vi "Command Run MP.vi"(7 "Startup":bool) -> (0 "Parameter 2":dbl, 1 "Parameter 1":dbl, 2 "Reinitialize":bool, 3 "Completed":bool)   [LabVIEW 2017]
uses:
  Command Execution State.ctl
  Drive/Drive Globals.vi
  Globals/Position Data.vi
  <vilib>/Utility/file.llb/Read Delimited Spreadsheet (DBL).vi
  <vilib>/Utility/file.llb/Read Delimited Spreadsheet (string).vi
panel:
  out "thetaError PID":T1(graph)
  in  "Path name":string
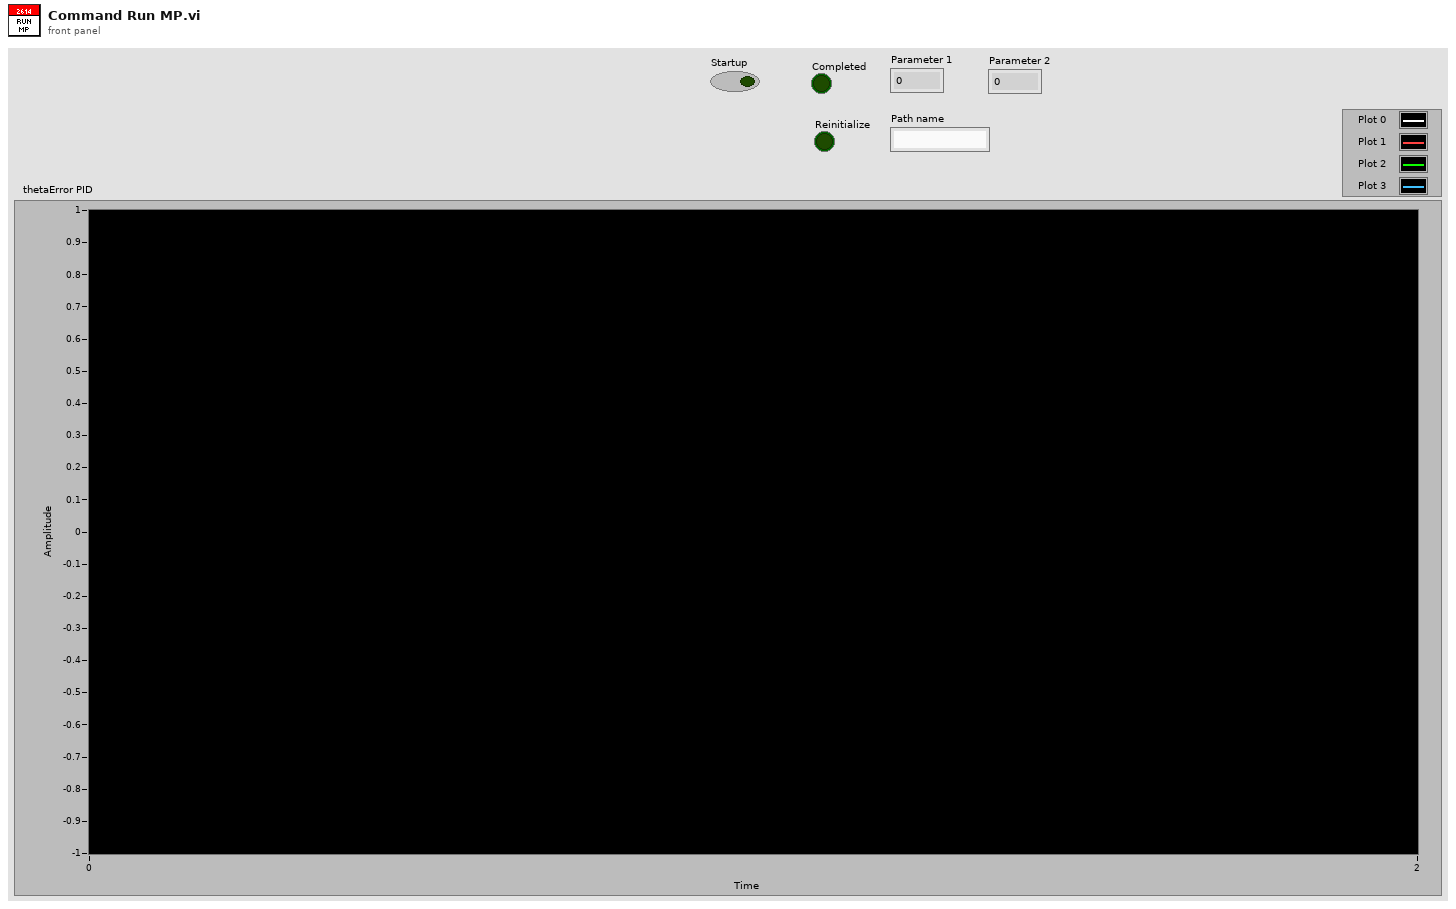
[diagram p1: front panel]
types:
  T1 = cluster{"Goal Wheel Position":dbl, dbl, "thetaError":dbl, "Command ":dbl}
  T2 = typedef "Command Execution State.ctl" = enum16{"Initialize", "Execute", "Finish"}
  T3 = cluster{"Goal Wheel Position":dbl, dbl, "Command ":dbl, "thetaError":dbl}
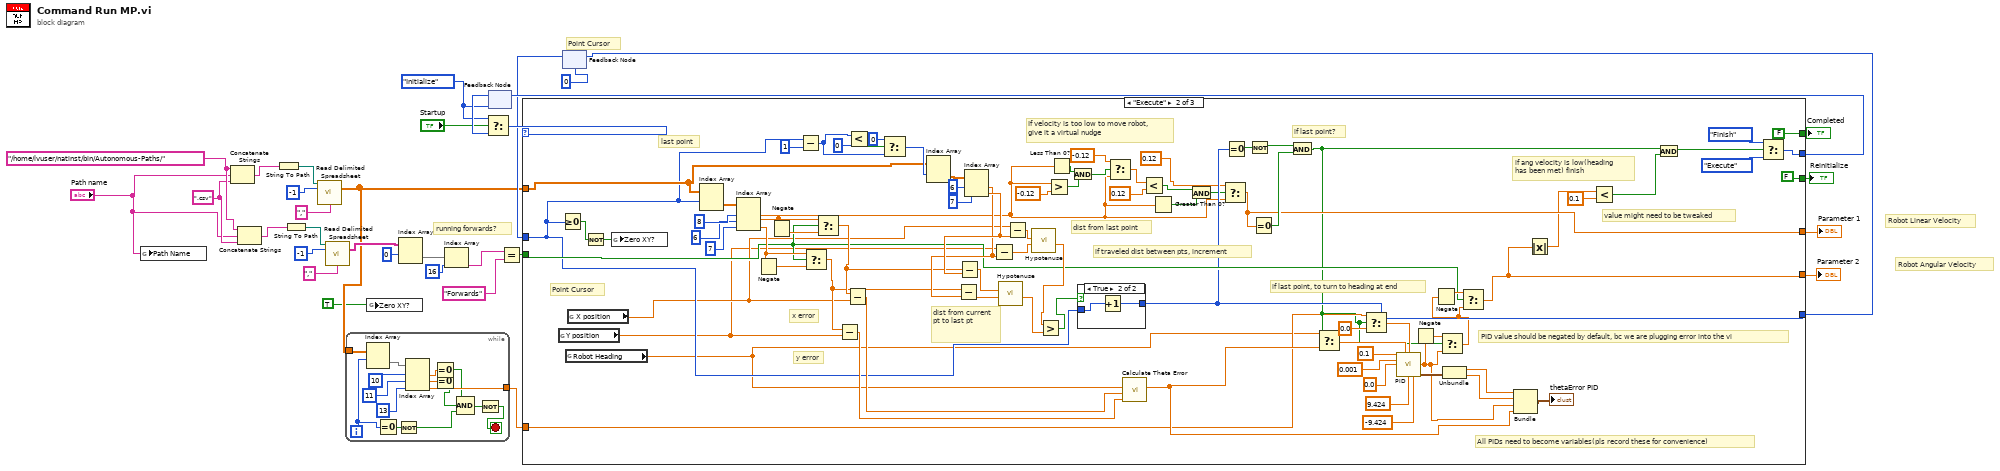
[diagram p0: block diagram]
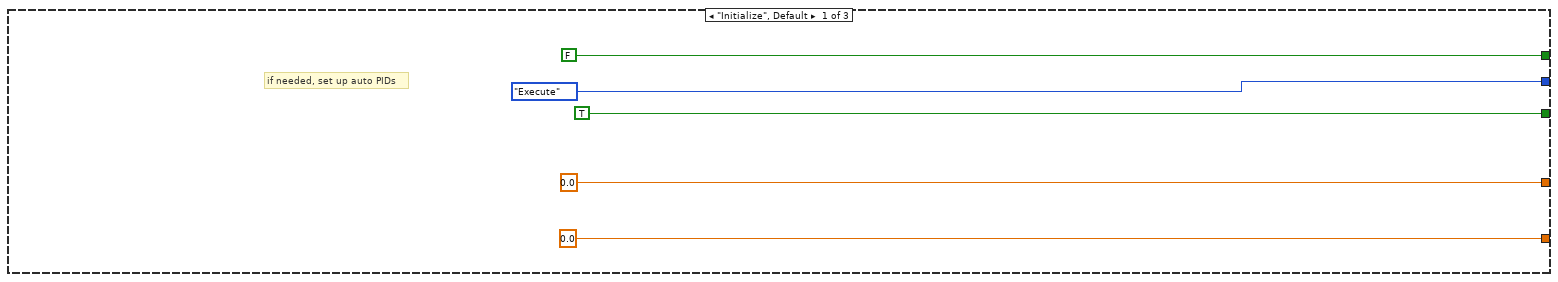
[diagram p2: hidden frame]
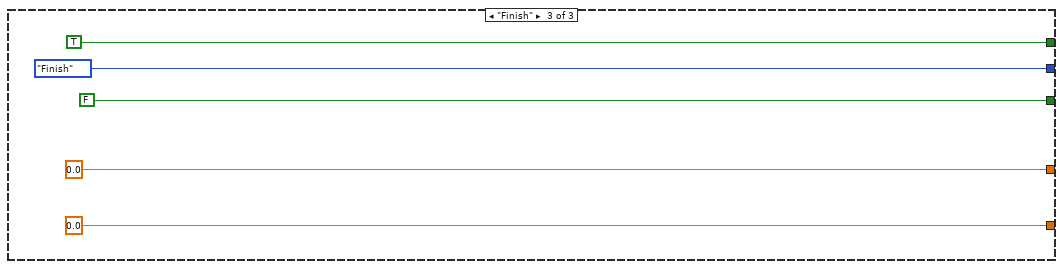
[diagram p4: hidden frame]
diagram:
  w12 = ".csv" ("string")
  w13 = "/home/lvuser/natinst/bin/Autonomous-Paths/"
  w28 = Command_Execution_State."Initialize" ("Play State")
  # "Point Cursor"
  # "running forwards?"
  # "Robot Angular Velocity"
  # "Robot Linear Velocity"
  n1 = global write "Position Data.vi" "Path Name"("Path name") -> ()
  n2 = Concatenate Strings(w13, "Path name", w12) -> (w22:string)
  n3 = Concatenate Strings(w13, "Path name", w12) -> (w16:string)
  n4 = String To Path(string=w22) -> (path=w21:path)
  n5 = String To Path(string=w16) -> (path=w17:path)
  n6 = call-poly <vilib>:"Read Delimited Spreadsheet.vi"("file path (dialog if empty)"=w21, "number of rows (all:-1)"=-1, "delimiter (\\t)"="," ("delimiter (\\t)")) -> ("all rows"=w3:dbl[][])  [unwired: 7 in, 5 out]
  n7 = call-poly <vilib>:"Read Delimited Spreadsheet.vi"("file path (dialog if empty)"=w17, "number of rows (all:-1)"=-1, "delimiter (\\t)"="," ("delimiter (\\t)")) -> ("all rows"=w11:string[][])  [unwired: 7 in, 5 out]
  n8 = while {
    tunnel: w3 -> [w48]
    tunnel: [w43] -> w2
    i -> [w40]
    stop <- w34 stop-if-true
    n9 = Index Array(array=w48, index (row)=w40) -> (element=w47:dbl[])  [unwired: 1 in]
    n10 = Equal To 0?(x=w40) -> (x = 0?=w39:bool)
    n11 = Not(x=w39) -> (.not. x?=w36:bool)
    n12 = Index Array(array=w47, index #1=10 ("index"), index #2=11 ("index"), index #3=13 ("index")) -> (element #1=w41:dbl, element #2=w42:dbl, element #3=w43:dbl)
    n13 = Equal To 0?(x=w41) -> (x = 0?=w37:bool)
    n14 = Equal To 0?(x=w42) -> (x = 0?=w38:bool)
    n15 = Compound Arithmetic op=AND(w37, w38, w36) -> (w35:bool)
    n16 = Not(x=w35) -> (.not. x?=w34:bool)
  }
  n17 = global write "Drive Globals.vi" "Zero XY?"(TRUE ("Zero XY?")) -> ()
  n18 = Index Array(array=w11, index (row)=0) -> (element=w20:string[])  [unwired: 1 in]
  n19 = Index Array(array=w20, index=16) -> (element=w10:string)
  n20 = feedback #1(w28) -> (w31:T2)
  n21 = Select(t=w28, s="Startup", f=w31) -> (s? t:f=w33:T2)
  n22 = Equal?(x=w10, y="Forwards") -> (x = y?=w8:bool)
  n23 = feedback #2(0 ("index")) -> (w6:i32)
  n24 = case shown="\"Execute\"" w33 {
    tunnel: [Command_Execution_State."Execute" ("Play State") w137 Command_Execution_State."Finish" ("Play State")] -> w32
    tunnel: [0.0 ("Back Left Spin Power") w72 0.0 ("Back Left Spin Power")] -> w30
    tunnel: [0.0 ("Front Right Spin Power") w63 0.0 ("Front Right Spin Power")] -> w29
    tunnel: [FALSE FALSE TRUE] -> w27
    tunnel: [TRUE FALSE FALSE] -> w26
    tunnel: w3 -> [_ w103 _]
    tunnel: w8 -> [_ w101 _]
    tunnel: w6 -> [_ w87 _]
    tunnel: [_ w85 _] -> w5
    tunnel: w2 -> [_ w68 _]
    frame "Initialize", Default {
      # "if needed, set up auto PIDs"
    }
    frame "Execute" {
      # "value might need to be tweaked"
      # "if ang velocity is low(heading\nhas been met) finish"
      # "if last point, to turn to heading at end"
      # "if last point?"
      # "PID value should be negated by default, bc we are plugging error into the vi"
      # "If velocity is too low to move robot,\ngive it a virtual nudge"
      # "if traveled dist between pts, increment"
      # "All PIDs need to become variables(pls record these for convenience)"
      # "dist from current pt to last pt"
      # "dist from last point"
      # "last point"
      # "y error"
      # "x error"
      # "Point Cursor"
      n25 = global read "Drive Globals.vi" "Y position"() -> (w54:dbl)
      n26 = Greater Or Equal To 0?(x=w87) -> (x >= 0?=w86:bool)
      n27 = global read "Drive Globals.vi" "Robot Heading"() -> (w56:dbl)
      n28 = global read "Drive Globals.vi" "X position"() -> (w55:dbl)
      n29 = Not(x=w86) -> (.not. x?=w57:bool)
      n30 = global write "Drive Globals.vi" "Zero XY?"(w57) -> ()
      n31 = Index Array(array=w103, index (row)=w87) -> (element=w132:dbl[])  [unwired: 1 in]
      n32 = Index Array(array=w132, index #1=8 ("index"), index #2=6 ("index"), index #3=7 ("index")) -> (element #1=w73:dbl, element #2=w108:dbl, element #3=w106:dbl)
      n33 = Negate(x=w106) -> (-x=w105:dbl)
      n34 = Negate(x=w108) -> (-x=w107:dbl)
      n35 = Subtract(x=w87, y=1) -> (x-y=w88:i32)
      n36 = Select(t=w106, s=w101, f=w105) -> (s? t:f=w104:dbl)
      n37 = Select(t=w108, s=w101, f=w107) -> (s? t:f=w109:dbl)
      n38 = Subtract(x=w104, y=w54) -> (x-y=w111:dbl)
      n39 = Subtract(x=w109, y=w55) -> (x-y=w110:dbl)
      n40 = Less?(x=w88, y=0) -> (x < y?=w115:bool)
      n41 = Select(t=0, s=w115, f=w88) -> (s? t:f=w112:i32)
      n42 = Index Array(array=w103, index (row)=w112) -> (element=w128:dbl[])  [unwired: 1 in]
      n43 = Index Array(array=w128, index #1=6 ("index"), index #2=7 ("index")) -> (element #1=w124:dbl, element #2=w125:dbl)
      n44 = Subtract(x=w104, y=w124) -> (x-y=w120:dbl)
      n45 = Subtract(x=w109, y=w125) -> (x-y=w121:dbl)
      n46 = Subtract(x=w54, y=w124) -> (x-y=w122:dbl)
      n47 = call "Hypotenuse.vi"("b"=w120, "a"=w121) -> ("c"=w119:dbl)  [unwired: 9 in]
      n48 = Subtract(x=w55, y=w125) -> (x-y=w123:dbl)
      n49 = call "Hypotenuse.vi"("b"=w122, "a"=w123) -> ("c"=w118:dbl)  [unwired: 9 in]
      n50 = Greater?(x=w118, y=w119) -> (0:w117:bool)
      n51 = Greater?(x=w73, y=-0.12) -> (0:w78:bool)
      n52 = Less Than 0?(x=w73) -> (x < 0?=w82:bool)
      n53 = And(x=w82, y=w78) -> (x .and. y?=w76:bool)
      n54 = case shown="True" w117 {
        tunnel: [w138 w140] -> w85
        tunnel: w87 -> [w138 w139]
        frame False {
        }
        frame True {
          n55 = Increment(x=w139) -> (x+1=w140:i32)
        }
      }
      n56 = Select(t=-0.12, s=w76, f=w73) -> (s? t:f=w75:dbl)
      n57 = call "Calculate Theta Error.vi"("yError"=w111, "xError"=w110, "heading"=w56) -> ("thetaError"=w71:dbl)  [unwired: 8 in]
      n58 = Less?(x=w75, y=0.12) -> (x < y?=w80:bool)
      n59 = Greater Than 0?(x=w73) -> (x > 0?=w81:bool)
      n60 = And(x=w80, y=w81) -> (x .and. y?=w79:bool)
      n61 = Select(t=0.12, s=w79, f=w73) -> (s? t:f=w72:dbl)
      n62 = Equal To 0?(x=w85) -> (x = 0?=w91:bool)
      n63 = Not(x=w91) -> (.not. x?=w89:bool)
      n64 = Equal To 0?(x=w72) -> (x = 0?=w90:bool)
      n65 = And(x=w89, y=w90) -> (x .and. y?=w58:bool)
      n66 = Select(t=w56, s=w58, f=w71) -> (s? t:f=w70:dbl)
      n67 = Select(t=w68, s=w58, f=0.0 ("Goal")) -> (s? t:f=w67:dbl)
      n68 = call "PID.vi"("Kp"=0.1, "Process Variable"=w70, "Goal"=w67, "Ki"=0.001, "Kd"=0.0, "Max Ouput"=9.424 ("x"), "Min Output"=-9.424 ("x")) -> ("Command"=w65:dbl, "PID Tracking"=w92:cluster{"Goal Wheel Position":dbl, dbl})  [unwired: 6 in, 1 out]
      n69 = Negate(x=w65) -> (-x=w64:dbl)
      n70 = Select(t=w64, s=w58, f=w65) -> (s? t:f=w66:dbl)
      n71 = Negate(x=w66) -> (-x=w102:dbl)
      n72 = Unbundle(w92) -> ("Goal Wheel Position"=w94:dbl, w95:dbl)
      n73 = Select(t=w102, s=w101, f=w66) -> (s? t:f=w63:dbl)
      n74 = Bundle("Goal Wheel Position"=w94, w95, "Command"=w65, "thetaError"=w71) -> (→"thetaError PID":T3)  [unwired: 1 in]
      n75 = Absolute Value(x=w63) -> (abs(x)=w62:dbl)
      n76 = Less?(x=w62, y=0.1) -> (x < y?=w59:bool)
      n77 = And(x=w58, y=w59) -> (x .and. y?=w60:bool)
      n78 = Select(t=Command_Execution_State."Finish" ("Play State"), s=w60, f=Command_Execution_State."Execute" ("Play State")) -> (s? t:f=w137:T2)
    }
    frame "Finish" {
    }
  }
  "Parameter 1" <- w30
  "Parameter 2" <- w29
  "Completed" <- w27
  "Reinitialize" <- w26
  n79 = feedback-in #1(w32) -> ()
  n80 = feedback-in #2(w5) -> ()
